vi "DetectorSelectionToString(SubVI).vi"(0 "Detector 1":bool, 1 "Detector 2":bool, 2 "Detector 3":bool, 3 "Detector 4":bool, 4 "Detector 5":bool, 5 "Detector 6":bool) -> (16 "Output strting":string)   [LabVIEW 2017]
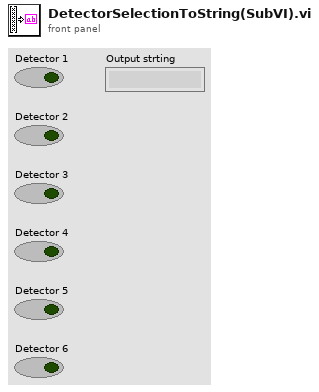
[diagram p1: front panel]
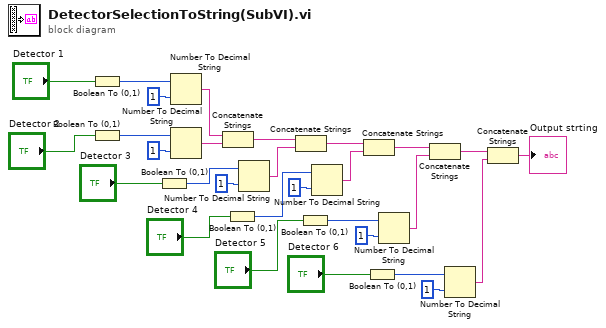
[diagram p0: block diagram]
diagram:
  n1 = Boolean To (0,1)(Boolean="Detector 1") -> (0, 1=w4:i16)
  n2 = Boolean To (0,1)(Boolean="Detector 2") -> (0, 1=w11:i16)
  n3 = Boolean To (0,1)(Boolean="Detector 3") -> (0, 1=w14:i16)
  n4 = Number To Decimal String(number=w4, width (-)=i16 1) -> (decimal integer string=w5:string)
  n5 = Number To Decimal String(number=w11, width (-)=i16 1) -> (decimal integer string=w12:string)
  n6 = Concatenate Strings(w5, w12) -> (w22:string)
  n7 = Boolean To (0,1)(Boolean="Detector 4") -> (0, 1=w16:i16)
  n8 = Number To Decimal String(number=w14, width (-)=i16 1) -> (decimal integer string=w21:string)
  n9 = Concatenate Strings(w22, w21) -> (w24:string)
  n10 = Boolean To (0,1)(Boolean="Detector 5") -> (0, 1=w18:i16)
  n11 = Number To Decimal String(number=w16, width (-)=i16 1) -> (decimal integer string=w23:string)
  n12 = Concatenate Strings(w24, w23) -> (w26:string)
  n13 = Boolean To (0,1)(Boolean="Detector 6") -> (0, 1=w20:i16)
  n14 = Number To Decimal String(number=w18, width (-)=i16 1) -> (decimal integer string=w25:string)
  n15 = Concatenate Strings(w26, w25) -> (w28:string)
  n16 = Number To Decimal String(number=w20, width (-)=i16 1) -> (decimal integer string=w27:string)
  n17 = Concatenate Strings(w28, w27) -> (→"Output strting":string)
